vi "Configure Setpoints Trim Limits.vi"(7 "Unit Address (1)":u8=1, 8 "error in (no error)":errorcluster, 9 "Setpoint Trim Limit Value (0)":i16, 10 "Enable Limit Type (False: High)":bool, 11 "VISA resource name":refnum<visa-resource-name>) -> (0 "error out":errorcluster, 3 "VISA resource name out":refnum<visa-resource-name>)   [LabVIEW 2014, in "Eurotherm 35xx Series.lvlib"]
doc: "This VI sets the Setpoints trim limits."
uses:
  <instrlib>/Eurotherm 35xx Series/Eurotherm 35xx Series.lvlib
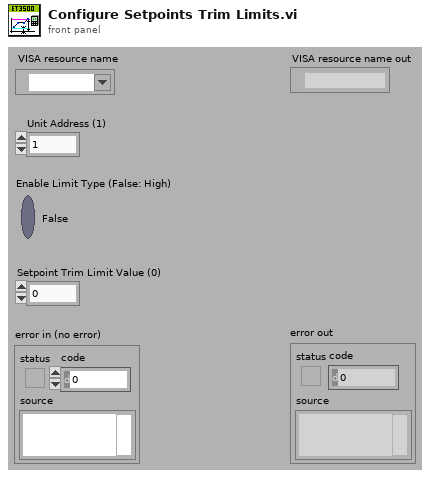
[diagram p1: front panel]
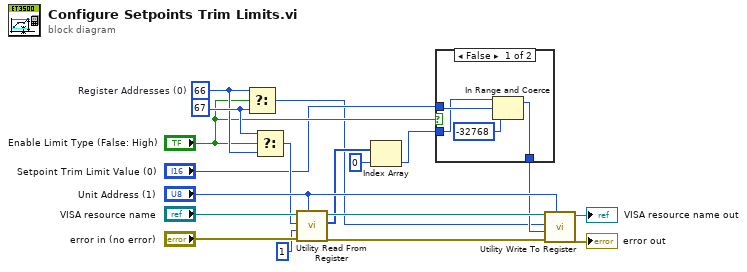
[diagram p0: block diagram]
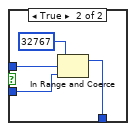
[diagram p2: hidden frame]
diagram:
  w10 = 67 ("Register Addresses (0)")
  w9 = 66  # Register Addresses (0)
  n1 = Select(t=w9, s="Enable Limit Type (False: High)", f=w10) -> (s? t:f=w1:i32)
  n2 = Select(t=w10, s="Enable Limit Type (False: High)", f=w9) -> (s? t:f=w8:i32)
  n3 = call <instrlib>:"Utility Read From Register.vi"("Unit Address (1)"="Unit Address (1)", "error in (no error)"="error in (no error)", "Num Of Reg (1)"=u16 1, "Register Address (0)"=w8, "VISA resource name"="VISA resource name") -> ("error out"=w14:errorcluster, "Data"=w7:i16[], "VISA resource name out"=w15:refnum<visa-resource-name>)  [unwired: 4 in]
  n4 = Index Array(array=w7, index=0) -> (element=w4:i16)
  n5 = case shown="False" "Enable Limit Type (False: High)" {
    tunnel: w4 -> [w20 w25]
    tunnel: "Setpoint Trim Limit Value (0)" -> [w22 w24]
    tunnel: [w19 w23] -> w2
    frame False {
      n6 = In Range and Coerce(upper limit=w20, x=w22, lower limit=-32768 ("upper limit")) -> (coerced(x)=w19:i32)  [unwired: 1 out]
    }
    frame True {
      n7 = In Range and Coerce(upper limit=32767, x=w24, lower limit=w25) -> (coerced(x)=w23:i32)  [unwired: 1 out]
    }
  }
  n8 = call <instrlib>:"Utility Write To Register.vi"("Unit Address (1)"="Unit Address (1)", "error in (no error)"=w14, "Data (0)"=w2, "Register Address (0)"=w1, "VISA resource name"=w15) -> ("error out"=→"error out":errorcluster, "VISA resource name out"=→"VISA resource name out":refnum<visa-resource-name>)  [unwired: 5 in]
